vi "Read value (String).vi"(8 "error in (no error)":errorcluster, 9 "default value":string, 11 "JSON String in":refnum<class "JSON Value.lvclass">) -> (0 "error out":errorcluster, 1 "defaulted?":bool, 2 "value":string)   [LabVIEW 2016, in "JSON Value.lvclass"]
doc: "Returns the value of a JSON String"
uses:
  JSON Value.lvclass
  JSON Value.lvclass/JSON Value.ctl
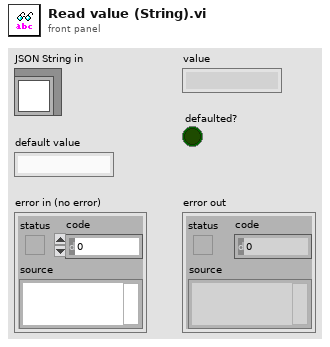
[diagram p1: front panel]
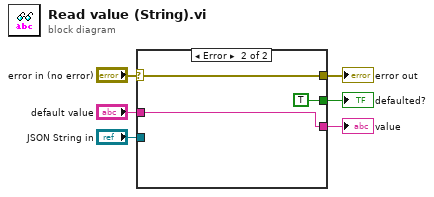
[diagram p0: block diagram]
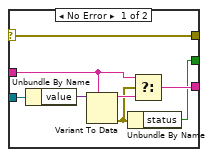
[diagram p2: hidden frame]
diagram:
  n1 = case shown="Error" "error in (no error)" {
    selector: "error in (no error)" -> [w14 w17]
    tunnel: [w14 w17] -> w5
    tunnel: "JSON String in" -> [w13 _]
    tunnel: [w9 w16] -> w3
    tunnel: "default value" -> [w11 w16]
    tunnel: [w7 TRUE ("status")] -> w1
    frame No Error {
      n2 = Unbundle By Name(w13) -> ("value"=w12:variant)
      n3 = Variant To Data(type=w11, Variant=w12) -> (data=w10:string, error out=w8:errorcluster)  [unwired: 1 in]
      n4 = Unbundle By Name(w8) -> ("status"=w7:bool)
      n5 = Select(t=w11, s=w8, f=w10) -> (s? t:f=w9:string)
    }
    frame Error {
    }
  }
  "error out" <- w5
  "value" <- w3
  "defaulted?" <- w1
